vi "gap_bw_twonums.vi"(0 "Y":dbl[](array[numeric]), 5 "element 1":dbl, 7 "element 2":dbl, 9 "length":i32, 11 "index":i32) -> (4 "Numeric":i32, 10 "element 2":dbl, 15 "element 1":dbl)   [LabVIEW 2023]
doc: "Used to find the number of element between two values in an array"
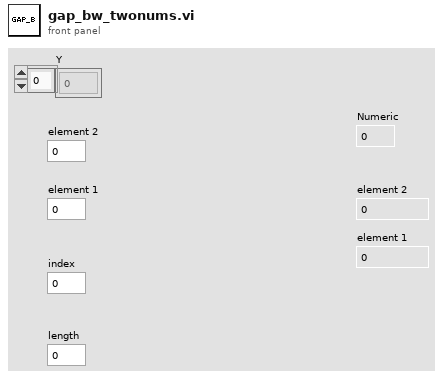
[diagram p1: front panel]
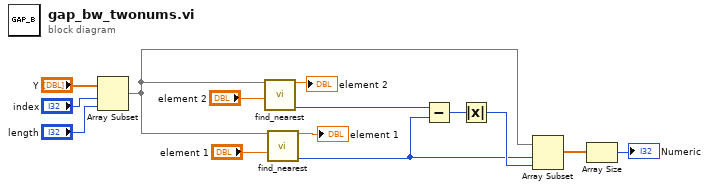
[diagram p0: block diagram]
diagram:
  n1 = Array Subset(array="Y", index="index", length="length") -> (w1:dbl[])
  n2 = call "find_nearest.vi"("Array"=w1, "element"="element 2") -> ("nearest element"=→"element 2":dbl, "min index(es)"=w8:i32)  [unwired: 12 in]
  n3 = call "find_nearest.vi"("Array"=w1, "element"="element 1") -> ("nearest element"=→"element 1":dbl, "min index(es)"=w5:i32)  [unwired: 12 in]
  n4 = Subtract(x=w8, y=w5) -> (x-y=w2:i32)
  n5 = Absolute Value(x=w2) -> (abs(x)=w9:i32)
  n6 = Array Subset(array=w1, index=w5, length=w9) -> (w3:dbl[])
  n7 = Array Size(array=w3) -> (size(s)=→"Numeric":i32)
